vi "HEWH Temp_In_Range.vi"(0 "MW100":refnum<visa-resource-name>, 2 "Semiphore":T1, 5 "upper limit":dbl=60.0, 7 "lower limit":dbl=56.0, 11 "Error In":errorcluster) -> (4 "Temp Value":dbl, 6 "In Range?":bool, 15 "Error Out":errorcluster={"status"=TRUE, "code"=1, "source"="Temperature Out of Range"})   [LabVIEW 2009]
uses:
  ChannelSettings.ctl
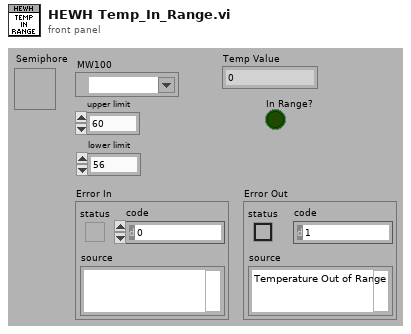
[diagram p1: front panel]
types:
  T1 = typedef "Semaphore RefNum" = refnum<k1>
  T2 = typedef "ChannelSettings.ctl" = u32
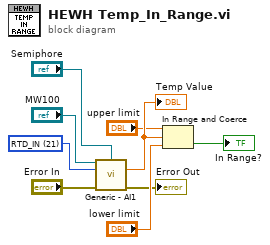
[diagram p0: block diagram]
diagram:
  w9 = T2 21 items=["4-20_OUT", "Pres_HI1", "Pres_HI2", "Pres_LOW", "Pres_PIN", "HEATER_TOP", "HEATER_BOT", "T_Shell", "FLOWMETER", "WATT_SENSE", "WH_TICK", "Tc_1", "Tc_2", "Tc_3", "Tc_4", "Tc_5", "Tc_6", "Tc_down", "T_Shell_2", "T_Shell_3", "T_Shell_4", "RTD_IN", "RTD_OUT", "RTD_AMB", "INTF_TEMPFLO", "INTF_READY", "INTF_START", "INTF_STOP", "DRM_LOW", "DRM_HIGH", "PWR_MAIN", "VLV_DUMP", "VLV_OUT", "VLV_IN", "WATT_HOURS", "FLOW(SAMPLE)", "GALLONS", "FLOW(GPM)"] ("Channel_Enum")
  n1 = call "Generic - AI1.vi"("MW100"="MW100", "Semiphore"="Semiphore", "Channel_Enum"=w9, "Error In"="Error In") -> ("Value"=w8:dbl, "Error Out"=→"Error Out":errorcluster)  [unwired: 9 in, 1 out]
  "Temp Value" <- w8
  n2 = In Range and Coerce(upper limit="upper limit", x=w8, lower limit="lower limit") -> (In Range?=→"In Range?":bool)  [unwired: 1 out]
